vi "Plot Format 2D Graph.vi"(6 "SYS|Plot|Unit":string, 8 "TBL1D":cluster{"X":sgl[], "Y":sgl[]}, 11 "XYGraph in":refnum<vi>) -> ()   [LabVIEW 2016]
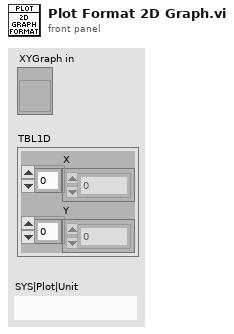
[diagram p1: front panel]
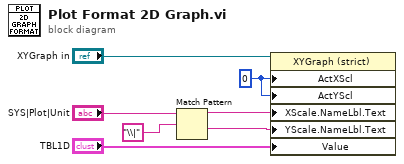
[diagram p0: block diagram]
diagram:
  w7 = 0 ("Active X Scale")
  n1 = Match Pattern(string="SYS|Plot|Unit", regular expression="\\|") -> (before substring=w2:string, after substring=w1:string)  [unwired: 1 in, 2 out]
  n2 = property on="Property Node" class="XYGraph (strict)"(reference="XYGraph in", "ActXScl"=w7, "ActYScl"=w7, "XScale.NameLbl.Text"=w2, "YScale.NameLbl.Text"=w1, "Value"="TBL1D") -> ()  [unwired: 1 in, 2 out]
